vi "Stop Task.vi"(8 "error in":errorcluster, 11 "NI Analog Output in":refnum<class "NI Analog Output.lvclass">) -> (0 "error out":errorcluster, 3 "NI Analog Output out":refnum<class "NI Analog Output.lvclass">)   [LabVIEW 2023, in "HardwareAbstractionLayer_LVOOP.lvlib" / "NI Analog Output.lvclass"]
doc: "This VI is DAQmx Stop the Task"
uses:
  NI Analog Output.lvclass
  NI Analog Output.lvclass/NI Analog Output.ctl
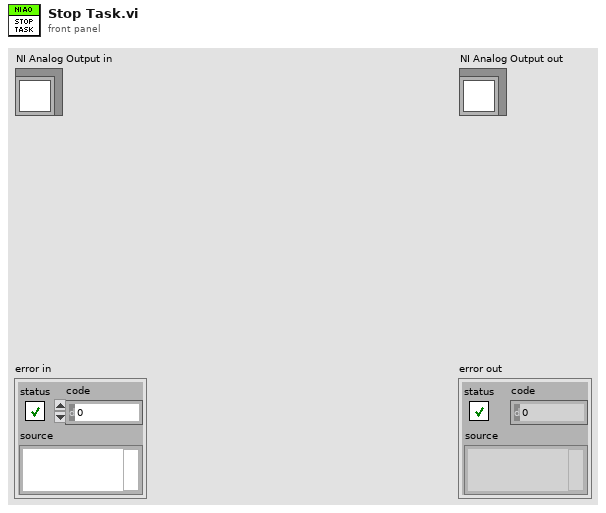
[diagram p1: front panel]
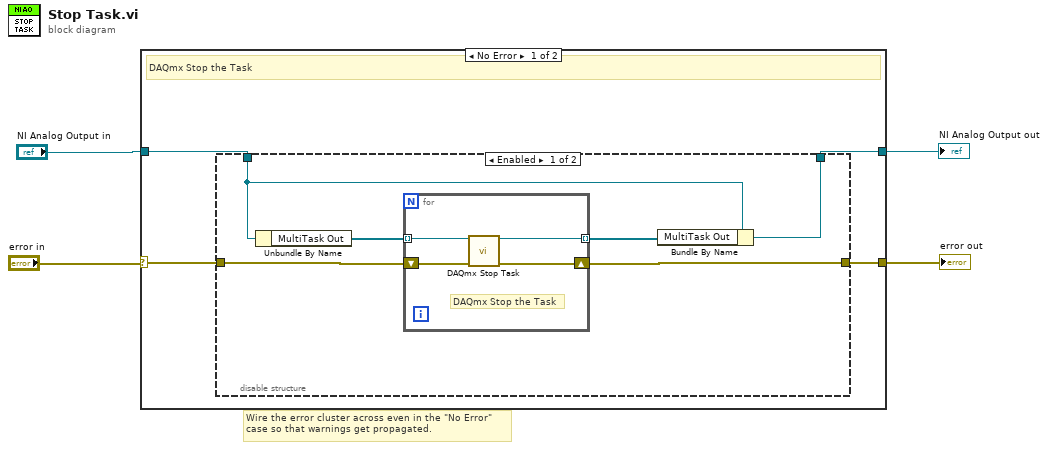
[diagram p0: block diagram]
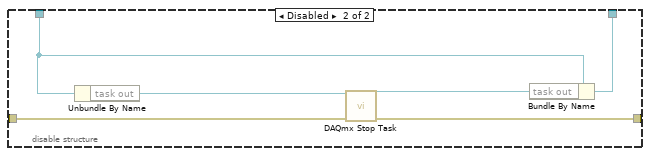
[diagram p2: hidden frame]
diagram:
  # "Wire the error cluster across even in the \"No Error\"\ncase so that warnings get propagated."
  n1 = case shown="No Error" "error in" {
    selector: "error in" -> [w8 w26]
    tunnel: [w7 w26] -> w3
    tunnel: [w5 w25] -> w1
    tunnel: "NI Analog Output in" -> [w6 w25]
    frame No Error {
      # "DAQmx Stop the Task"
      n2 = disable-structure shown="Enabled" {
        disable-tunnel: w8 -> [w14 w23]
        disable-tunnel: [w13 w22] -> w7
        disable-tunnel: w6 -> [w11 w21]
        disable-tunnel: [w10 w20] -> w5
        frame Enabled {
          n3 = Unbundle By Name(w11) -> ("MultiTask Out"=w12:refnum<k21>[])
          n4 = for {
            shift-right: [w17] -> w13
            shift-left: w14 -> [w18]
            tunnel: w12 -> [w16] mode=indexing
            tunnel: [w15] -> w9 mode=indexing
            # "DAQmx Stop the Task"
            n5 = call <vilib>:"DAQmx Stop Task.vi"("task/channels in"=w16, "error in"=w18) -> ("task out"=w15:refnum<k21>, "error out"=w17:errorcluster)  [unwired: 12 in]
          }
          n6 = Bundle By Name(cluster=w11, "MultiTask Out"=w9) -> (w10:refnum<class "NI Analog Output.lvclass">)
        }
        frame Disabled {
          n7 = Unbundle By Name(w21) -> ("task out"=w24:refnum<k21>)
          n8 = call <vilib>:"DAQmx Stop Task.vi"("task/channels in"=w24, "error in"=w23) -> ("task out"=w19:refnum<k21>, "error out"=w22:errorcluster)  [unwired: 12 in]
          n9 = Bundle By Name(cluster=w21, "task out"=w19) -> (w20:refnum<class "NI Analog Output.lvclass">)
        }
      }
    }
    frame Error {
    }
  }
  "error out" <- w3
  "NI Analog Output out" <- w1
